vi "GT Start Handwheel.vi"(0 "cardNum":i16, 1 "slaveEven":i16, 2 "acc":dbl, 3 "vel":dbl, 5 "slave":i16, 7 "master":i16, 9 "masterEven":i16, 11 "error in (no error)":errorcluster caption="错误输入（无错误）", 12 "intervalTime":i16, 13 "dec":dbl, 14 "stopWaitTime":i16) -> (4 "function return":i16, 15 "error out":errorcluster caption="错误输出")   [LabVIEW 2014, in "gts.lvlib"]
doc: "GT_API GT_StartHandwheel(short cardNum,short slave,short master,short masterEven,short slaveEven,short intervalTime,double acc,double dec,double vel,short stopWaitTime);"
uses:
  gts.lvlib
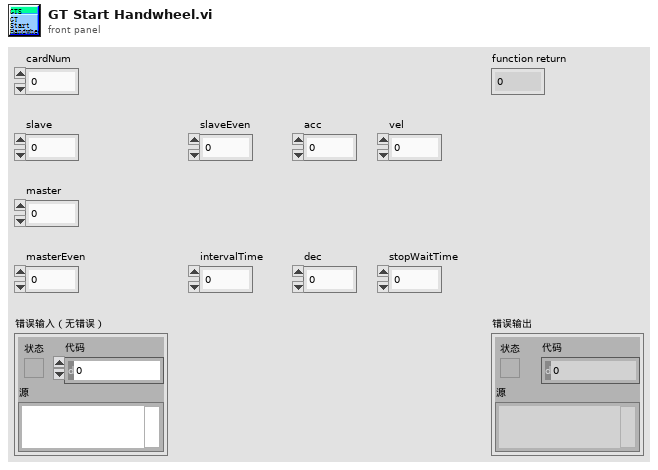
[diagram p1: front panel]
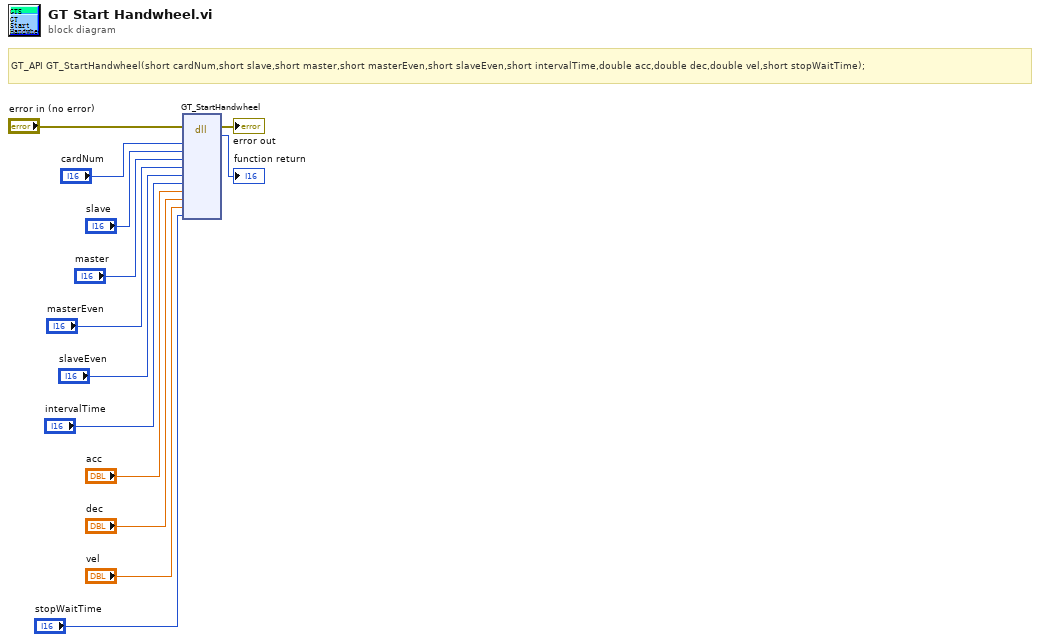
[diagram p0: block diagram]
diagram:
  # "GT_API GT_StartHandwheel(short cardNum,short slave,short master,short masterEven,short slaveEven,short intervalTime,double acc,double dec,double vel,short stopWaitTime);"
  n1 = dll-call lib="PTH2habs D固高科技资料GTS控制卡GTS卡18年上半年资料dllVC32bit\nmulti_cardgts.*" fn="GT_StartHandwheel"(error in="error in (no error)", "cardNum"="cardNum", "slave"="slave", "master"="master", "masterEven"="masterEven", "slaveEven"="slaveEven", "intervalTime"="intervalTime", "acc"="acc", "dec"="dec", "vel"="vel", "stopWaitTime"="stopWaitTime") -> (error out=→"error out":errorcluster, →"function return":i16)  [unwired: 12 in, 1 out]
